vi "Menu_Create.vi"(8 "Error In":errorcluster, 9 "Description":string, 10 "Name":string, 11 "reference in":refnum<class "Menu.lvclass">) -> (0 "Error Out":errorcluster, 3 "reference out":refnum<class "Menu.lvclass">)   [LabVIEW 2020, in "Menu.lvclass"]
uses:
  Menu.lvclass
  C:/Projects/DesignPatterns/Composition/MenuComponent_class/MenuComponent.lvclass
  MenuComponent_class/MenuComponent.lvclass
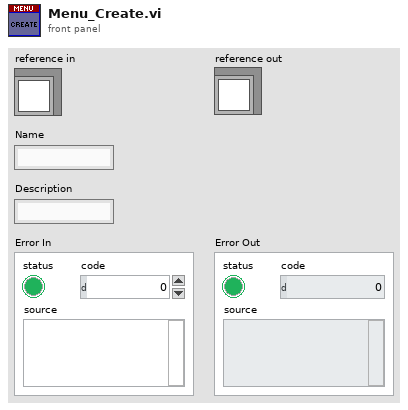
[diagram p1: front panel]
types:
  T1 = typedef "Menu.lvclass/ObjectAttributes.ctl" = cluster{"Items":refnum<class "MenuComponent.lvclass">[], "Name":string, "Description":string}
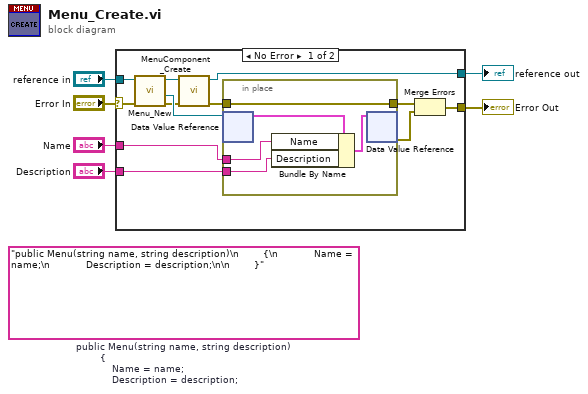
[diagram p0: block diagram]
diagram:
  (unwired) "public Menu(string name, string description)\n        {\n            Name = name;\n            Description = description;\n\n        }"  # public Menu(string name, string description)         {             Name = name;             Description = description;          }
  n1 = case shown="No Error" "Error In" {
    selector: "Error In" -> [w14 w25]
    tunnel: [w12 w25] -> w5
    tunnel: "reference in" -> [w16 w24]
    tunnel: [w11 w24] -> w3
    tunnel: "Name" -> [w8 _]
    tunnel: "Description" -> [w7 _]
    frame No Error {
      n2 = call "Menu_New.vi"("error in (no error)"=w14, "reference in"=w16) -> ("error out"=w15:errorcluster, "DVRRefOut"=w18:refnum<data-value>, "reference out"=w17:refnum<class "Menu.lvclass">)  [unwired: 6 in, 1 out]
      n3 = call "MenuComponent_Create.vi"("Error In"=w15, "reference in"=w17) -> ("Error Out"=w10:errorcluster, "reference out"=w11:refnum<class "Menu.lvclass">)  [unwired: 8 in]
      n4 = in-place {
        in-place-border: w10 -> [w21]
        in-place-border: [w21] -> w9
        in-place-border: w8 -> [w20]
        in-place-border: w7 -> [w19]
        n5 = in-place-dvr #1(w18) -> (w22:T1)  [unwired: 1 out]
        n6 = Bundle By Name(cluster=w22, "Name"=w20, "Description"=w19) -> (w23:T1)
        n7 = in-place-dvr #1(w23) -> (w13:errorcluster)  [unwired: 1 out]
      }
      n8 = Merge Errors(w9, w13) -> (w12:errorcluster)
    }
    frame Error {
    }
  }
  "Error Out" <- w5
  "reference out" <- w3
